vi "Add Seconds.vi"(6 "reset minute?":bool, 10 "seconds":dbl, 11 "time in":dbl format="%<%H:%M:%S>t") -> (3 "time out":dbl format="%<%H:%M:%S>t")   [LabVIEW 2019, in "Pet Feeder.lvlib"]
uses:
  Pet Feeder.lvlib
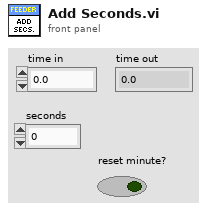
[diagram p1: front panel]
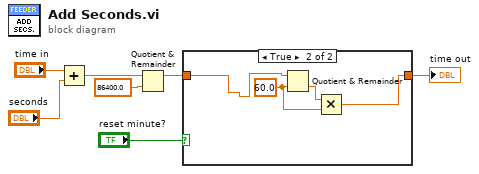
[diagram p0: block diagram]
diagram:
  n1 = Add(x="time in", y="seconds") -> (x+y=w6:dbl)
  n2 = Quotient & Remainder(x=w6, y=86400.0) -> (x-y*floor(x/y)=w1:dbl)  [unwired: 1 out]
  n3 = case shown="True" "reset minute?" {
    tunnel: w1 -> [w8 w9]
    tunnel: [w8 w10] -> w3
    frame False {
    }
    frame True {
      w11 = 60.0 ("y")
      n4 = Quotient & Remainder(x=w9, y=w11) -> (floor(x/y)=w12:dbl)  [unwired: 1 out]
      n5 = Multiply(x=w12, y=w11) -> (x*y=w10:dbl)
    }
  }
  "time out" <- w3
